vi "S2DS_Users latest info (SubVI).vi"(8 "error in (no error)":errorcluster, 10 "User name":string) -> (0 "Email":string, 1 "Latest session":string, 2 "Latest project":string, 3 "File prefix":string, 4 "error out":errorcluster, 5 "Project list":string[](array[string]), 7 "Logbook path":path)   [LabVIEW 2025]
uses:
  <vilib>/Utility/config.llb/Read Key (I32).vi
  <vilib>/Utility/config.llb/Read Key (String).vi
  <vilib>/Utility/config.llb/Read Key (Path).vi
  <vilib>/Utility/config.llb/NI_LVConfig.lvlib
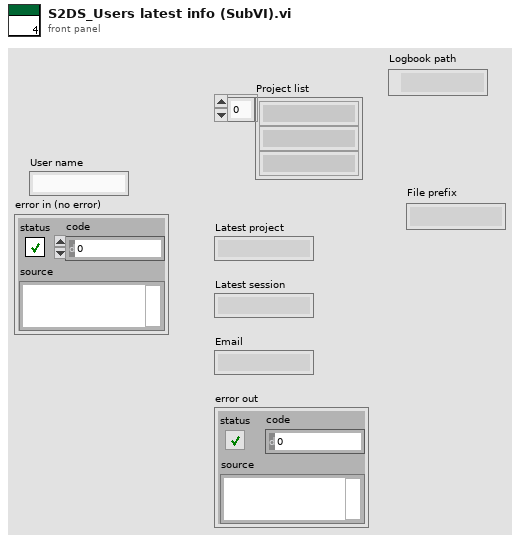
[diagram p1: front panel]
types:
  T1 = typedef "NI_LVConfig.lvlib/Config Data RefNum.ctl" = refnum<k1>
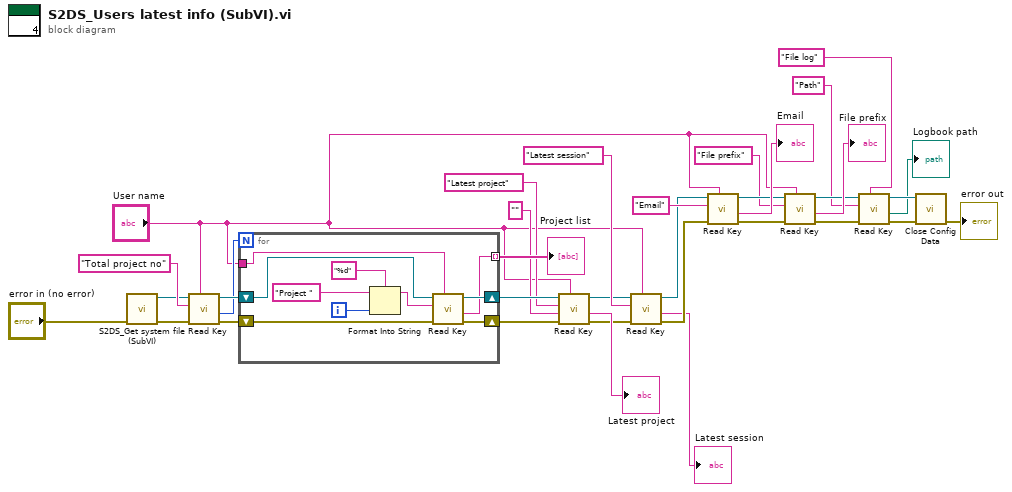
[diagram p0: block diagram]
diagram:
  n1 = call "S2DS_Get system file (SubVI).vi"("error in (no error)"="error in (no error)") -> ("error out"=w16:errorcluster, "Refnum out"=w15:T1)  [unwired: 9 in]
  n2 = call-poly <vilib>:"Read Key.vi"("section"="User name", "error in (no error)"=w16, "key"="Total project no", "refnum"=w15) -> ("error out"=w25:errorcluster, "value"=w23:i32, "refnum out"=w24:T1)  [unwired: 4 in, 1 out]
  n3 = for {
    N: w23 -> [_]
    shift-right: [w41] -> w29
    shift-left: w24 -> [w44]
    shift-right: [w42] -> w30
    shift-left: w25 -> [w43]
    tunnel: "User name" -> [w40]
    tunnel: [w35] -> w26 mode=indexing
    i -> [w36]
    n4 = Format Into String(format string="%d", initial string="Project ", w36) -> (resulting string=w38:string)  [unwired: 1 in, 1 out]
    n5 = call-poly <vilib>:"Read Key.vi"("section"=w40, "error in (no error)"=w43, "key"=w38, "refnum"=w44) -> ("error out"=w42:errorcluster, "value"=w35:string, "refnum out"=w41:T1)  [unwired: 4 in, 1 out]
  }
  "Project list" <- w26
  n6 = call-poly <vilib>:"Read Key.vi"("section"="User name", "error in (no error)"=w30, "default value"="", "key"="Latest project", "refnum"=w29) -> ("error out"=w19:errorcluster, "value"=→"Latest project":string, "refnum out"=w20:T1)  [unwired: 3 in, 1 out]
  n7 = call-poly <vilib>:"Read Key.vi"("section"="User name", "error in (no error)"=w19, "key"="Latest session", "refnum"=w20) -> ("error out"=w33:errorcluster, "value"=→"Latest session":string, "refnum out"=w31:T1)  [unwired: 4 in, 1 out]
  n8 = call-poly <vilib>:"Read Key.vi"("section"="User name", "error in (no error)"=w33, "key"="Email", "refnum"=w31) -> ("error out"=w11:errorcluster, "value"=→"Email":string, "refnum out"=w12:T1)  [unwired: 4 in, 1 out]
  n9 = call-poly <vilib>:"Read Key.vi"("section"="User name", "error in (no error)"=w11, "key"="File prefix", "refnum"=w12) -> ("error out"=w6:errorcluster, "value"=→"File prefix":string, "refnum out"=w7:T1)  [unwired: 4 in, 1 out]
  n10 = call-poly <vilib>:"Read Key.vi"("section"="File log", "error in (no error)"=w6, "key"="Path", "refnum"=w7) -> ("error out"=w5:errorcluster, "value"=→"Logbook path":path, "refnum out"=w4:T1)  [unwired: 4 in, 1 out]
  n11 = call <vilib>:"Close Config Data.vi"("error in (no error)"=w5, "refnum"=w4) -> ("error out"=→"error out":errorcluster)  [unwired: 8 in, 1 out]
